vi "Write Output Data.vi"(10 "Output Data":T1, 11 "TestDataLog in":refnum<class "TestDataLog.lvclass">) -> (3 "TestDataLog out":refnum<class "TestDataLog.lvclass">)   [LabVIEW 2013, in "TestDataLog.lvclass"]
uses:
  TestDataLog.lvclass
  Typedefs/OutputData.ctl
  TestDataLog.lvclass/TestDataLog.ctl
  Typedefs/ILCBTTypedefs.lvlib
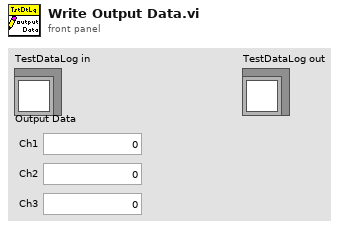
[diagram p1: front panel]
types:
  T1 = typedef "ILCBTTypedefs.lvlib/OutputData.ctl" = cluster{"Ch1":u16, "Ch2":u16, "Ch3":u16}
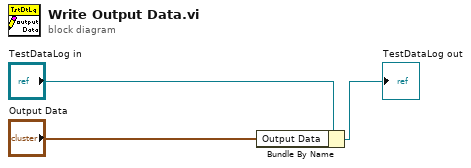
[diagram p0: block diagram]
diagram:
  n1 = Bundle By Name(cluster="TestDataLog in", "Output Data"="Output Data") -> (→"TestDataLog out":refnum<class "TestDataLog.lvclass">)
